vi "AOtrigger.vi"() -> ()   [LabVIEW 2018]
doc: "This example demonstrates how to generate a finite amount of digital data based off of a sample clock.\n\nSome hardware (e.g. M Series DAQ) must use an external sample clock for digital tasks. To view a complete list of available sample clock sources, consult the Device Routes table in Measurement and Automation Explorer.\n\nFor instructions on how to connect your signals to the DAQ device, refer to your device documentation."
uses:
  <vilib>/DAQmx/write.llb/DAQmx Write (Digital 1D U32 1Chan NSamp).vi
  <vilib>/DAQmx/create/channels.llb/DAQmx Create Channel (DO-Digital Output).vi
  <vilib>/DAQmx/miscellaneous.llb/DAQmx Fill In Error Info.vi
panel:
  in  "dimension size":i32
  in  "Count(uSec)":u32=50
  out "t2":u32=16016
  out "t3":u32=16072
  out "t1":u32=15925
  in  "Output Array":u32[](array[numeric])=[1, 0]
  in  "Line(s)":tag="6509/port1/line0"
  # "Channel Settings"
  # "Data to Write"
  # "6509, 6602, 6723, 6733\nall similar\n25-35 us to write\n300-500 us to clear"
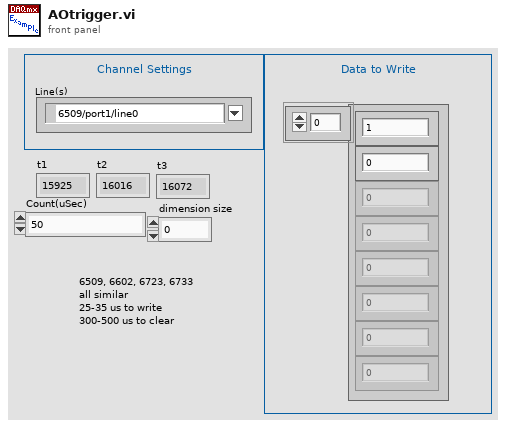
[diagram p1: front panel]
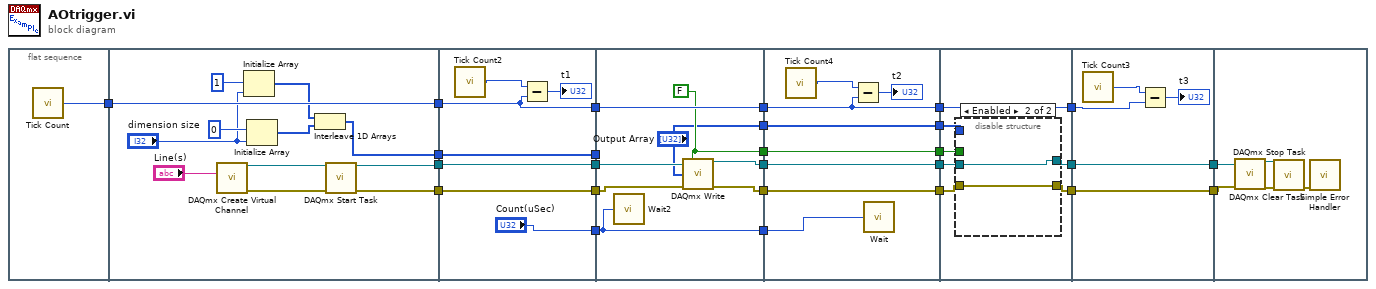
[diagram p0: block diagram]
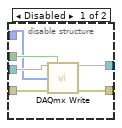
[diagram p2: hidden frame]
diagram:
  n1 = flat-sequence {
    tunnel: [w27] -> w24
    tunnel: [w36] -> w26
    tunnel: [w35] -> w25
    tunnel: w24 -> [w34]
    tunnel: [w34] -> w23
    tunnel: [w28] -> w1
    tunnel: w26 -> [w46]
    tunnel: w25 -> [w45]
    tunnel: w23 -> [w43]
    tunnel: [w46] -> w22
    tunnel: [w45] -> w21
    tunnel: [w43] -> w20
    tunnel: ["Count(uSec)"] -> w5
    tunnel: [w40] -> w2
    tunnel: w1 -> [w40]
    tunnel: w22 -> [w53]
    tunnel: [w52] -> w19
    tunnel: w21 -> [w50]
    tunnel: w20 -> [w54]
    tunnel: [w54] -> w18
    tunnel: [w51] -> w17
    tunnel: [w49] -> w10
    tunnel: ["Output Array"] -> w7
    tunnel: [w48] -> w6
    tunnel: w5 -> [w48]
    tunnel: w2 -> [_]
    tunnel: w19 -> [w62]
    tunnel: [w62] -> w16
    tunnel: [w61] -> w15
    tunnel: w18 -> [w60]
    tunnel: [w60] -> w13
    tunnel: w17 -> [w61]
    tunnel: w10 -> [w59]
    tunnel: [w59] -> w9
    tunnel: [w58] -> w8
    tunnel: w7 -> [w58]
    tunnel: w6 -> [w55]
    tunnel: w16 -> [w68]
    tunnel: w15 -> [w67]
    tunnel: [w66] -> w14
    tunnel: w13 -> [w69]
    tunnel: [w69] -> w12
    tunnel: [w65] -> w11
    tunnel: w9 -> [w64]
    tunnel: w8 -> [w63]
    tunnel: w14 -> [w80]
    tunnel: w12 -> [w82]
    tunnel: w11 -> [w81]
    tunnel: [w81] -> w4
    tunnel: [w80] -> w3
    tunnel: w4 -> [w84]
    tunnel: w3 -> [w83]
    frame #0 {
      n2 = call "Tick Count"() -> ("Tick Count(uSec)"=w27:u32)
    }
    frame #1 {
      n3 = call-poly <vilib>:"DAQmx Create Virtual Channel.vi"("lines"="Line(s)") -> ("task out"=w38:refnum<k21>, "error out"=w39:errorcluster)  [unwired: 13 in]
      n4 = Initialize Array(1, "dimension size") -> (w29:i32[])
      n5 = Initialize Array(0, "dimension size") -> (w30:i32[])
      n6 = Interleave 1D Arrays(w29, w30) -> (w28:i32[])
      n7 = call <vilib>:"DAQmx Start Task.vi"("task/channels in"=w38, "error in"=w39) -> ("task out"=w36:refnum<k21>, "error out"=w35:errorcluster)  [unwired: 12 in]
    }
    frame #2 {
      n8 = call "Tick Count2"() -> ("Tick Count(uSec)"=w42:u32)
      n9 = Subtract(x=w42, y=w43) -> (x-y=→"t1":u32)
    }
    frame #3 {
      w49 = FALSE ("auto start")
      n10 = call "Wait2"("Count(uSec)"=w48) -> ()  [unwired: 1 out]
      n11 = call-poly <vilib>:"DAQmx Write.vi"("task/channels in"=w53, "auto start"=w49, "data"="Output Array", "error in"=w50) -> ("task out"=w52:refnum<k21>, "error out"=w51:errorcluster)  [unwired: 9 in, 1 out]
    }
    frame #4 {
      n12 = call "Tick Count4"() -> ("Tick Count(uSec)"=w57:u32)
      n13 = Subtract(x=w57, y=w60) -> (x-y=→"t2":u32)
      n14 = call "Wait"("Count(uSec)"=w55) -> ()  [unwired: 1 out]
    }
    frame #5 {
      n15 = disable-structure shown="Enabled" {
        disable-tunnel: w68 -> [w75 w77]
        disable-tunnel: w67 -> [w74 w76]
        disable-tunnel: [w73 w76] -> w66
        disable-tunnel: [w72 w77] -> w65
        disable-tunnel: w64 -> [w71 _]
        disable-tunnel: w63 -> [w70 _]
        frame Disabled {
          n16 = call-poly <vilib>:"DAQmx Write.vi"("task/channels in"=w75, "auto start"=w71, "data"=w70, "error in"=w74) -> ("task out"=w72:refnum<k21>, "error out"=w73:errorcluster)  [unwired: 9 in, 1 out]
        }
        frame Enabled {
        }
      }
    }
    frame #6 {
      n17 = call "Tick Count3"() -> ("Tick Count(uSec)"=w79:u32)
      n18 = Subtract(x=w79, y=w82) -> (x-y=→"t3":u32)
    }
    frame #7 {
      n19 = call <vilib>:"DAQmx Stop Task.vi"("task/channels in"=w84, "error in"=w83) -> ("task out"=w86:refnum<k21>, "error out"=w85:errorcluster)  [unwired: 12 in]
      n20 = call <vilib>:"DAQmx Clear Task.vi"("task in"=w86, "error in"=w85) -> ("error out"=w87:errorcluster)  [unwired: 13 in]
      n21 = call <vilib>:"Simple Error Handler.vi"("error in (no error)"=w87) -> ()  [unwired: 4 in, 5 out]
    }
  }
